vi "F to C.vi"(10 "Value [°F]":dbl) -> (2 "Value [°C]":dbl)   [LabVIEW 2014, in "Dual Mode Thermometer.lvclass"]
doc: "Helper function to convert Farenheit to Celcius.\n\n\nCopyright (c) 2019 Sze Howe Koh.\nThis code is licensed under the MIT license."
uses:
  Dual Mode Thermometer.lvclass
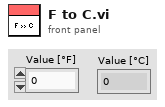
[diagram p1: front panel]
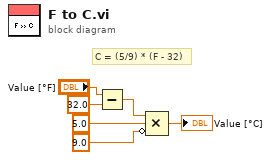
[diagram p0: block diagram]
diagram:
  # "C = (5/9) * (F - 32)"
  n1 = Subtract(x="Value [°F]", y=32.0) -> (x-y=w4:dbl)
  n2 = Compound Arithmetic op=MULTIPLY(w4, 5.0 ("value"), invert 9.0 ("value")) -> (→"Value [°C]":dbl)
